vi "Serial Read for Arduino with Control.vi"() -> ()   [LabVIEW 2024]
doc: "This example performs writes and reads on a serial port, as directed by the user. You can press the Write and Read buttons, and change the Read Count, while the example is running.\n\nThe parameters set for the serial port must match the parameters of the connected instrument or device. In this example, the Read Count parameter specifies the number of bytes that the serial port reads. If there were more bytes at the port than the specified number, those bytes would not be read. If there were less bytes at the port than the specified number, you would receive a timeout error.\n\nThis example expands upon the flow control options for XON and XOFF, allowing the user to choose those control characters. Also, the user can enable or disable a termination character. Some devices require a termination character in order to identify the end of command strings. Some devices send a termination character to signify the end of data to be read. This example shows how you can end the Read operation once a termination character is detected in the buffer and/or append a termination character at the end of the Write data."
uses:
  support/Serial - Settings.ctl
  <vilib>/Instr/_visa.llb/VISA Flush IO Buffer Mask.ctl
  <vilib>/Instr/_visa.llb/VISA Configure Serial Port (Instr).vi
panel:
  out "Raw Out Graph":dbl[][](graph)
  in  "Data Format":enum32{"Foece Mode", "Raw Mode"}(radio)=enum."Raw Mode"
  out "Raw":bool=TRUE
  out "Force":bool
  in  "Zero Reset":bool
  out "Foece Graph":dbl[][](graph)
  in  "Termination Character":u8=10 format="%.0x"
  in  "End Write on Termination Character?":bool=TRUE
  in  "Stop":bool
  in  "Serial Settings":T1={"baud rate"=115200, "data bits"=8, "parity"=enum."None", "stop bits"=10, "flow control"=0} {"flow control" items=["None"=0, "XON/XOFF"=1, "RTS/CTS"=2, "DTR/DSR"=4]; "stop bits" items=["1.0"=10, "1.5"=15, "2.0"=20]; "data bits" min=5 max=8 step=1; "baud rate" items=["75"=75, "110"=110, "134"=134, "150"=150, "300"=300, "600"=600, "1200"=1200, "1800"=1800, "2400"=2400, "4800"=4800, "7200"=7200, "9600"=9600, "14400"=14400, "19200"=19200, "28800"=28800, "38400"=38400, "56000"=56000, "57600"=57600, "115200"=115200, "128000"=128000, "230400"=230400]}
  in  "End Read on Termination Character?":bool=TRUE
  in  "VISA resource name":refnum<visa-resource-name>="COM1"
  # "Overview: Serial Based Data Viewer\n\nSet COM Port before start IV\nInitial mode is RAW mode. \nIgnore  radio burron at start"
  # "0xA is equivalent to a '\\n' character, which is a line feed."
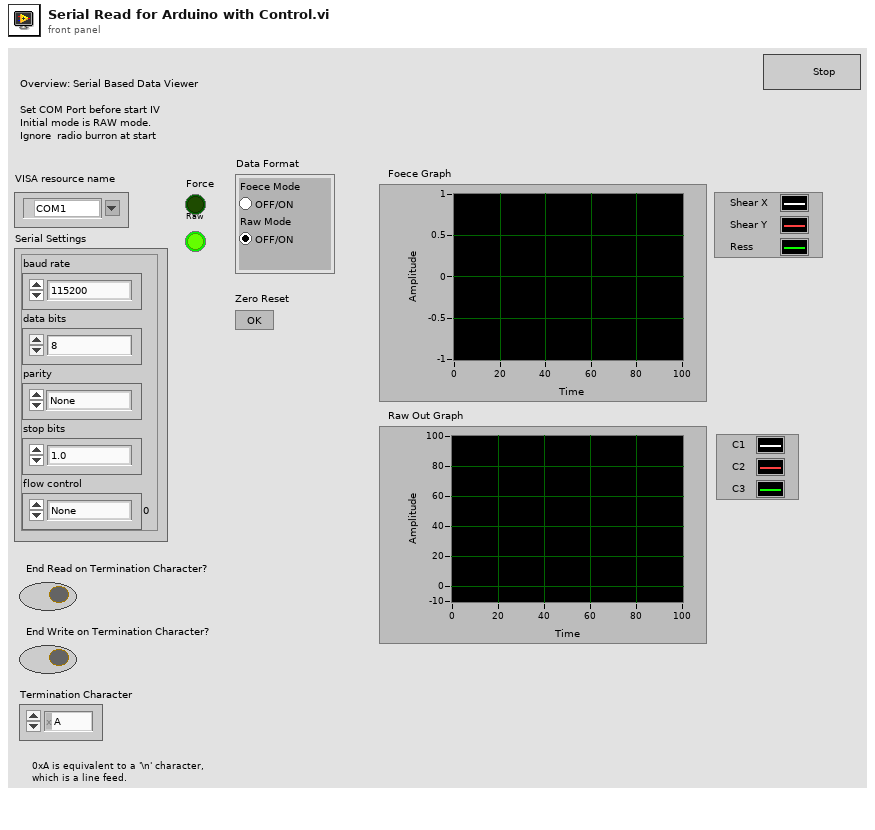
[diagram p1: front panel]
types:
  T1 = typedef "Serial - Settings.ctl" = cluster{"baud rate":u32, "data bits":u16, "parity":enum16{"None", "Odd", "Even", "Mark", "Space"}, "stop bits":u16, "flow control":u16}
  T2 = typedef "VISA Flush IO Buffer Mask.ctl" = u16
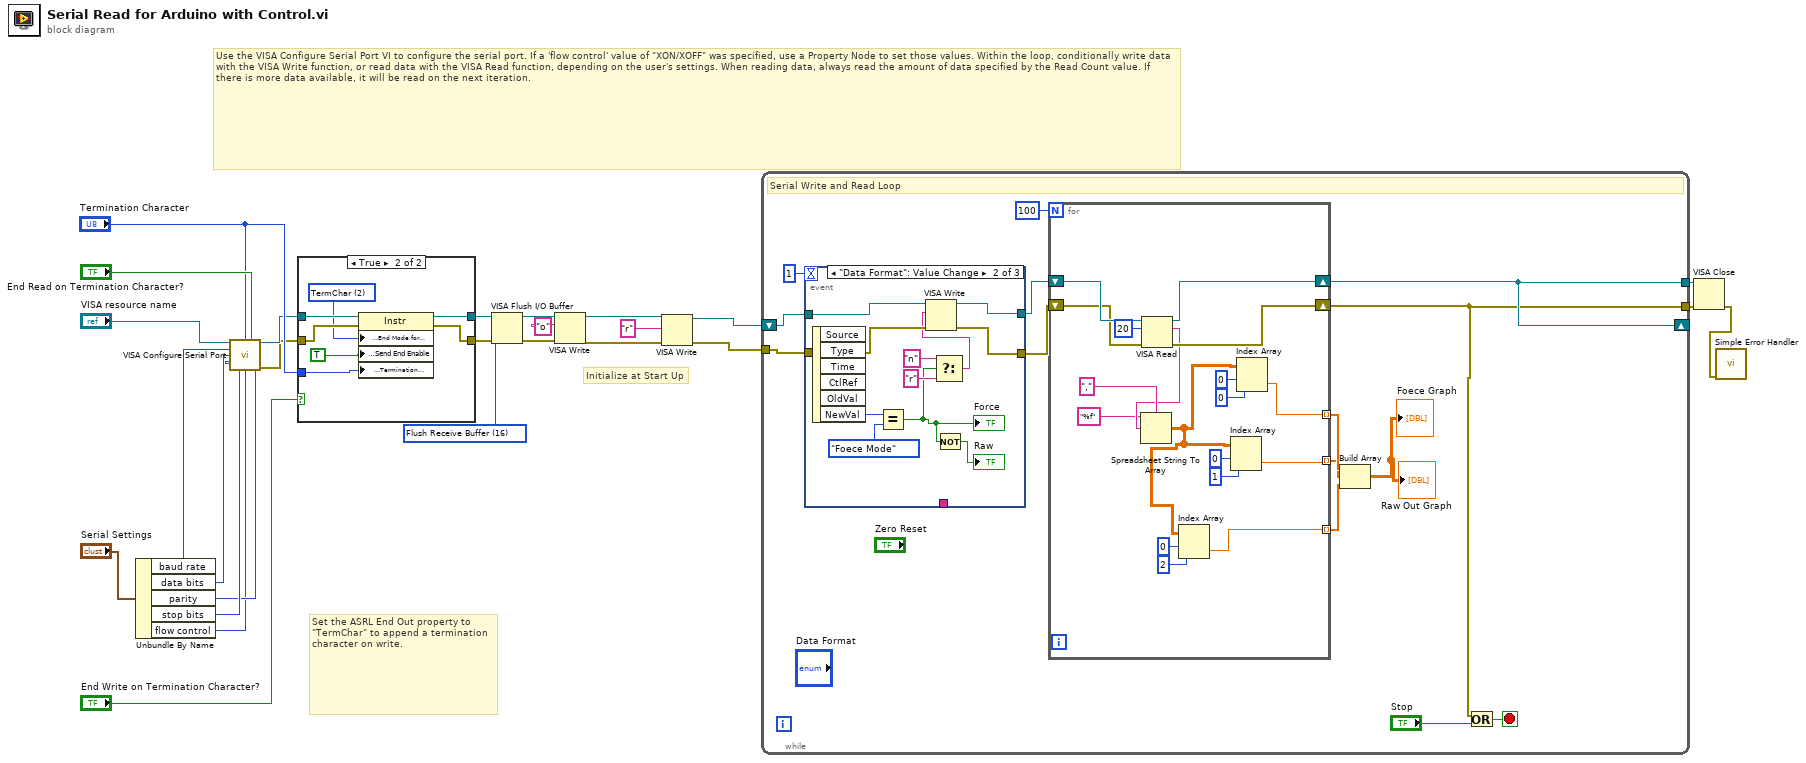
[diagram p0: block diagram]
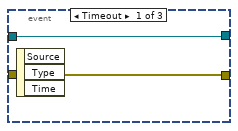
[diagram p3: hidden frame]
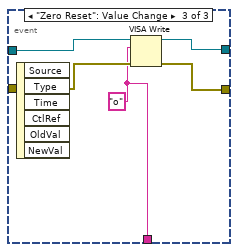
[diagram p4: hidden frame]
diagram:
  w9 = T2 16 items=["Flush Receive Buffer"=16, "Write Transmit Buffer to Device"=32, "Flush Receive Buffer (No I/O)"=64, "Flush Transmit Buffer"=128] ("Mask")
  # "Initialize at Start Up"
  # "Set the ASRL End Out property to \"TermChar\" to append a termination character on write."
  # "Use the VISA Configure Serial Port VI to configure the serial port. If a 'flow control' value of \"XON/XOFF\" was specified, use a Property Node to set those values. Within the loop, conditionally write data with the VISA Write function, or read data with the VISA Read function, depending on the user's settings. When reading data, always read the amount of data specified by the Read Count value. If there is more data available, it will be read on the next iteration."
  n1 = Unbundle By Name("Serial Settings") -> ("baud rate"=w22:u32, "data bits"=w23:u16, "parity"=w24:enum16{"None", "Odd", "Even", "Mark", "Space"}, "stop bits"=w25:u16, "flow control"=w19:u16)
  n2 = call-poly "VISA Configure Serial Port"("VISA resource name"="VISA resource name", "termination char\n(0xA = '\\n' = LF)"="Termination Character", "Enable Termination\nChar (T)"="End Read on Termination Character?", "baud rate (9600)"=w22, "data bits (8)"=w23, "parity (0:none)"=w24, "stop bits (10: 1 bit)"=w25, "flow control (0:none)"=w19) -> ("VISA resource name out"=w16:refnum<visa-resource-name>, "error out"=w15:errorcluster)  [unwired: 2 in, 4 out]
  n3 = case shown="True" "End Write on Termination Character?" {
    tunnel: w16 -> [w27 w35]
    tunnel: w15 -> [w28 w34]
    tunnel: [w27 w33] -> w11
    tunnel: [w28 w32] -> w10
    tunnel: "Termination Character" -> [_ w30]
    frame False {
    }
    frame True {
      w31 = u16 2 items=["None", "LastBit", "TermChar", "Break"] ("Serial Settings:Serial End Mode for Writes")
      n4 = property class="Instr"(reference=w35, error in=w34, "Serial Settings:End Mode for Writes"=w31, "Message Based Settings:Send End Enable"=TRUE, "Message Based Settings:Termination Character"=w30) -> (reference out=w33:refnum<visa-resource-name>, error out=w32:errorcluster)
    }
  }
  n5 = VISA Flush I/O Buffer(VISA resource name=w11, mask (16)=w9, error in (no error)=w10) -> (VISA resource name out=w8:refnum<visa-resource-name>, error out=w7:errorcluster)
  n6 = VISA Write(VISA resource name=w8, write buffer="o", error in (no error)=w7) -> (VISA resource name out=w5:refnum<visa-resource-name>, error out=w4:errorcluster)  [unwired: 1 out]
  n7 = VISA Write(VISA resource name=w5, write buffer="r", error in (no error)=w4) -> (VISA resource name out=w3:refnum<visa-resource-name>, error out=w2:errorcluster)  [unwired: 1 out]
  n8 = while {
    shift-right: [w47] -> _
    shift-left: w3 -> [w40]
    tunnel: w2 -> [w41]
    tunnel: [w46] -> w14
    tunnel: [w47] -> w13
    stop <- w49 stop-if-true
    # "Serial Write and Read Loop"
    n9 = event shown="[1] \"Data Format\": Value Change" {
      selector: _ -> [_ _ _]
      dyn-events: _ -> [_ _ _]
      timeout: 1 -> [_ _ _]
      tunnel: w41 -> [w50 w61 w67]
      tunnel: w40 -> [w51 w62 w66]
      tunnel: [w51 w59 w65] -> w39
      tunnel: [w50 w60 w64] -> w38
      tunnel: [_ _ w63] -> _
      event Timeout {
        n10 = event-data() -> ()  [unwired: 1 in, 3 out]
      }
      event "Data Format": Value Change {
        n11 = event-data() -> ("NewVal"=w57:enum32{"Foece Mode", "Raw Mode"})  [unwired: 1 in, 5 out]
        n12 = Equal?(x=w57, y=enum16{"Foece Mode", "Raw Mode", ""}."Foece Mode") -> (x = y?=w54:bool)
        "Force" <- w54
        n13 = Select(t="n", s=w54, f="r") -> (s? t:f=w52:string)
        n14 = VISA Write(VISA resource name=w62, write buffer=w52, error in (no error)=w61) -> (VISA resource name out=w59:refnum<visa-resource-name>, error out=w60:errorcluster)  [unwired: 1 out]
        n15 = Not(x=w54) -> (.not. x?=→"Raw":bool)
      }
      event "Zero Reset": Value Change {
        w63 = "o" ("write buffer")
        n16 = event-data() -> ()  [unwired: 1 in, 6 out]
        n17 = VISA Write(VISA resource name=w66, write buffer=w63, error in (no error)=w67) -> (VISA resource name out=w65:refnum<visa-resource-name>, error out=w64:errorcluster)  [unwired: 1 out]
      }
    }
    n18 = for {
      N: 100 -> [_]
      shift-right: [w82] -> w47
      shift-left: w39 -> [w85]
      shift-right: [w83] -> w46
      shift-left: w38 -> [w84]
      tunnel: [w74] -> w44 mode=indexing
      tunnel: [w73] -> w45 mode=indexing
      tunnel: [w69] -> w42 mode=indexing
      n19 = VISA Read(VISA resource name=w85, byte count=u32 20, error in (no error)=w84) -> (VISA resource name out=w82:refnum<visa-resource-name>, read buffer=w76:string, error out=w83:errorcluster)  [unwired: 1 out]
      n20 = Spreadsheet String To Array(delimiter (Tab)=",", format string="%f", spreadsheet string=w76) -> (array=w70:dbl[][])  [unwired: 1 in]
      n21 = Index Array(array=w70, index (row)=0, index (col)=2 ("disabled index (col)")) -> (element=w69:dbl)
      n22 = Index Array(array=w70, index (row)=0, index (col)=1 ("disabled index (col)")) -> (element=w74:dbl)
      n23 = Index Array(array=w70, index (row)=0, index (col)=0 ("disabled index (col)")) -> (element=w73:dbl)
    }
    n24 = Build Array(w45, w44, w42) -> (→"Foece Graph" →"Raw Out Graph":dbl[][])
    n25 = Or(x=w46, y="Stop") -> (x .or. y?=w49:bool)
  }
  n26 = VISA Close(VISA resource name=w13, error in (no error)=w14) -> (error out=w12:errorcluster)
  n27 = call <vilib>:"Simple Error Handler.vi"("error in (no error)"=w12) -> ()  [unwired: 1 in, 8 out]
